vi "ControlList.vi"() -> (0 "Tab Control":cluster{"Control Path":string, "Data":variant}[](array[cluster]), 1 "BigCluster":cluster{"Control Path":string, "Data":variant}[](array[cluster]), 2 "Cluster":cluster{"Control Path":string, "Data":variant}[](array[cluster]), 3 "Basic":cluster{"Control Path":string, "Data":variant}[](array[cluster]), 4 "SubPanel":cluster{"Control Path":string, "Data":variant}[](array[cluster]), 6 "BasicArray":cluster{"Control Path":string, "Data":variant}[](array[cluster]))   [LabVIEW 2016, in "DronaTest.lvlib"]
uses:
  DronaTest.lvlib
  TestHelper/controls/Level2.ctl
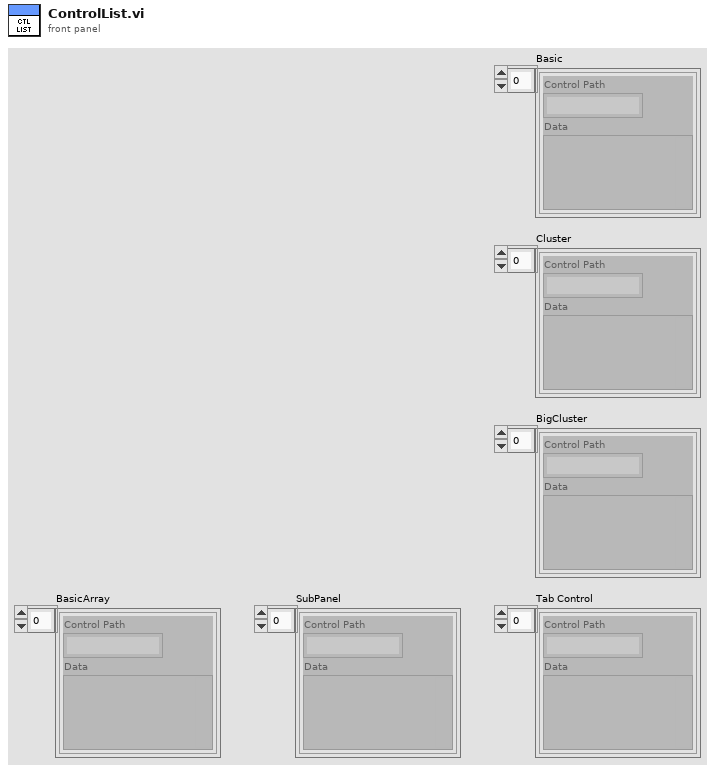
[diagram p1: front panel]
types:
  T1 = typedef "Level2.ctl" = cluster{"Numeric_cluster":dbl, "Boolean_cluster":bool, "target":string}
  T2 = cluster{"Control Path":string, "BigCluster":cluster{"Numeric_cluster":dbl, "Boolean_cluster":bool, "String_cluster":string, "Level1":cluster{"Numeric_cluster":dbl, "Boolean_cluster":bool, "String_cluster":string, "Level2":T1}}}
  T3 = cluster{"Control Path":string, "Data":cluster{"Numeric_cluster":dbl, "Boolean_cluster":bool, "String_cluster":string}}
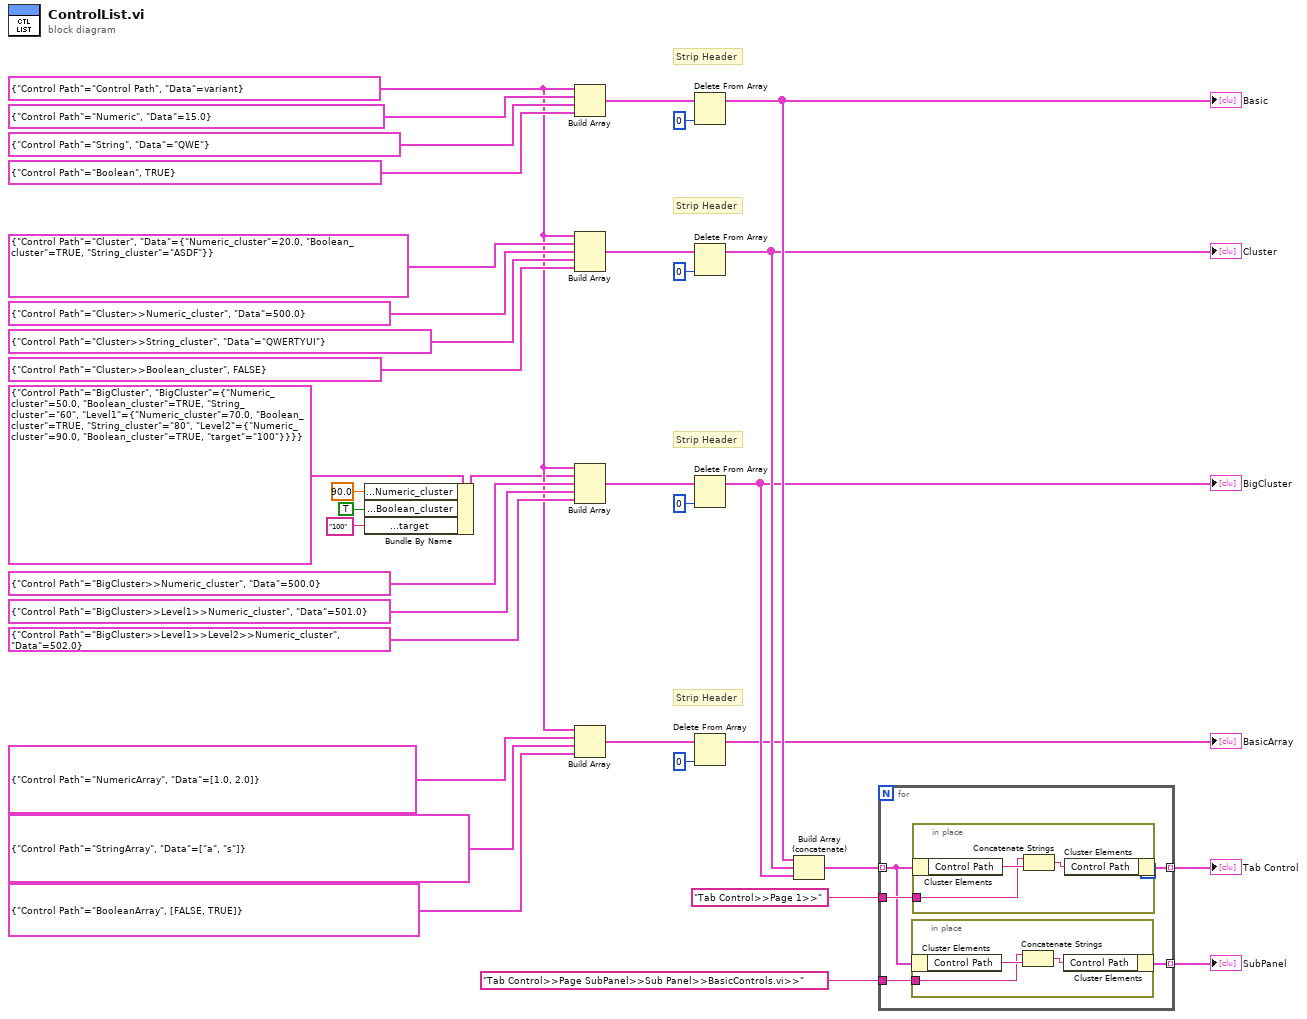
[diagram p0: block diagram]
diagram:
  w8 = cluster{"Control Path":string, "Data":variant} {"Control Path"="Control Path", "Data"=variant}
  # "Strip Header"
  # "Strip Header"
  # "Strip Header"
  # "Strip Header"
  n1 = Bundle By Name(cluster=T2 {"Control Path"="BigCluster", "BigCluster"={"Numeric_cluster"=50.0, "Boolean_cluster"=TRUE, "String_cluster"="60", "Level1"={"Numeric_cluster"=70.0, "Boolean_cluster"=TRUE, "String_cluster"="80", "Level2"={"Numeric_cluster"=90.0, "Boolean_cluster"=TRUE, "target"="100"}}}}, "BigCluster.Level1.Level2.Numeric_cluster"=90.0 ("Numeric_cluster"), "BigCluster.Level1.Level2.Boolean_cluster"=TRUE ("Boolean_cluster"), "BigCluster.Level1.Level2.target"="100" ("target")) -> (w4:T2)
  n2 = Build Array(w8, cluster{"Control Path":string, "Data":dbl} {"Control Path"="Numeric", "Data"=15.0}, cluster{"Control Path":string, "Data":string} {"Control Path"="String", "Data"="QWE"}, cluster{"Control Path":string, bool} {"Control Path"="Boolean", TRUE}) -> (w32:cluster{"Control Path":string, "Data":variant}[])
  n3 = Build Array(w8, T3 {"Control Path"="Cluster", "Data"={"Numeric_cluster"=20.0, "Boolean_cluster"=TRUE, "String_cluster"="ASDF"}}, cluster{"Control Path":string, "Data":dbl} {"Control Path"="Cluster>>Numeric_cluster", "Data"=500.0}, cluster{"Control Path":string, "Data":string} {"Control Path"="Cluster>>String_cluster", "Data"="QWERTYUI"}, cluster{"Control Path":string, bool} {"Control Path"="Cluster>>Boolean_cluster", FALSE}) -> (w26:cluster{"Control Path":string, "Data":variant}[])
  n4 = Build Array(w8, w4, cluster{"Control Path":string, "Data":dbl} {"Control Path"="BigCluster>>Numeric_cluster", "Data"=500.0}, cluster{"Control Path":string, "Data":dbl} {"Control Path"="BigCluster>>Level1>>Numeric_cluster", "Data"=501.0}, cluster{"Control Path":string, "Data":dbl} {"Control Path"="BigCluster>>Level1>>Level2>>Numeric_cluster", "Data"=502.0}) -> (w25:cluster{"Control Path":string, "Data":variant}[])
  n5 = Build Array(w8, cluster{"Control Path":string, "Data":dbl[]} {"Control Path"="NumericArray", "Data"=[1.0, 2.0]}, cluster{"Control Path":string, "Data":string[]} {"Control Path"="StringArray", "Data"=["a", "s"]}, cluster{"Control Path":string, bool[]} {"Control Path"="BooleanArray", [FALSE, TRUE]}) -> (w13:cluster{"Control Path":string, "Data":variant}[])
  n6 = Delete From Array(array=w32, index=0) -> (array with subset deleted=w19:cluster{"Control Path":string, "Data":variant}[])  [unwired: 1 in, 1 out]
  "Basic" <- w19
  n7 = Delete From Array(array=w26, index=0) -> (array with subset deleted=w18:cluster{"Control Path":string, "Data":variant}[])  [unwired: 1 in, 1 out]
  "Cluster" <- w18
  n8 = Delete From Array(array=w25, index=0) -> (array with subset deleted=w17:cluster{"Control Path":string, "Data":variant}[])  [unwired: 1 in, 1 out]
  "BigCluster" <- w17
  n9 = Delete From Array(array=w13, index=0) -> (array with subset deleted=→"BasicArray":cluster{"Control Path":string, "Data":variant}[])  [unwired: 1 in, 1 out]
  n10 = Build Array (concatenate)(w19, w18, w17) -> (w14:cluster{"Control Path":string, "Data":variant}[])
  n11 = for {
    tunnel: w14 -> [w39] mode=indexing
    tunnel: [w41] -> w15 mode=indexing
    tunnel: "Tab Control>>Page 1>>" ("Control Path") -> [w40]
    tunnel: "Tab Control>>Page SubPanel>>Sub Panel>>BasicControls.vi>>" ("Control Path") -> [w38]
    tunnel: [w37] -> w5 mode=indexing
    n12 = in-place {
      in-place-border: w38 -> [w42]
      n13 = in-place-cluster #1(w39) -> ("Control Path"=w43:string)
      n14 = Concatenate Strings(w42, w43) -> (w44:string)
      n15 = in-place-cluster #1("Control Path"=w44) -> (w37:cluster{"Control Path":string, "Data":variant})
    }
    n16 = in-place {
      in-place-border: w40 -> [w45]
      n17 = in-place-cluster #2(w39) -> ("Control Path"=w46:string)
      n18 = Concatenate Strings(w45, w46) -> (w47:string)
      n19 = in-place-cluster #2("Control Path"=w47) -> (w41:cluster{"Control Path":string, "Data":variant})
    }
  }
  "Tab Control" <- w15
  "SubPanel" <- w5
